vi "ConnectTestDisconnect.vi"() -> ()   [LabVIEW 2019]
panel:
  in  "DropPlate":u32=3229614090
  in  "Operation":T1(ring)
  in  "Autofocus":bool
  out "error out":errorcluster
  out "Image 2":T2(plugin-control)
  out "BestZvalue":dbl
  out "GantryXYUsingCamXY":cluster{"XmmGH":dbl, "YmmGH":dbl}
  in  "CamPixels":T3
  out "LogFilesPath":path
  in  "JoyStick":bool
  in  "GetHeightGauge Status":bool
  out "HeightGaugeTouch":bool
  out "SDofHeight(mm)":dbl format="%0.3f"
  out "MeanHeight(mm)":dbl format="%0.3f"
  in  "DistSensor":bool
  out "Position_XYZ":string
  in  "GetGantryXYZ":bool
  in  "DropTool":i32
  in  "PickPlate":u32=3233808386
  in  "PickTool":u32=3229614090
  in  "Z":dbl=50.0
  in  "PickDrop":bool
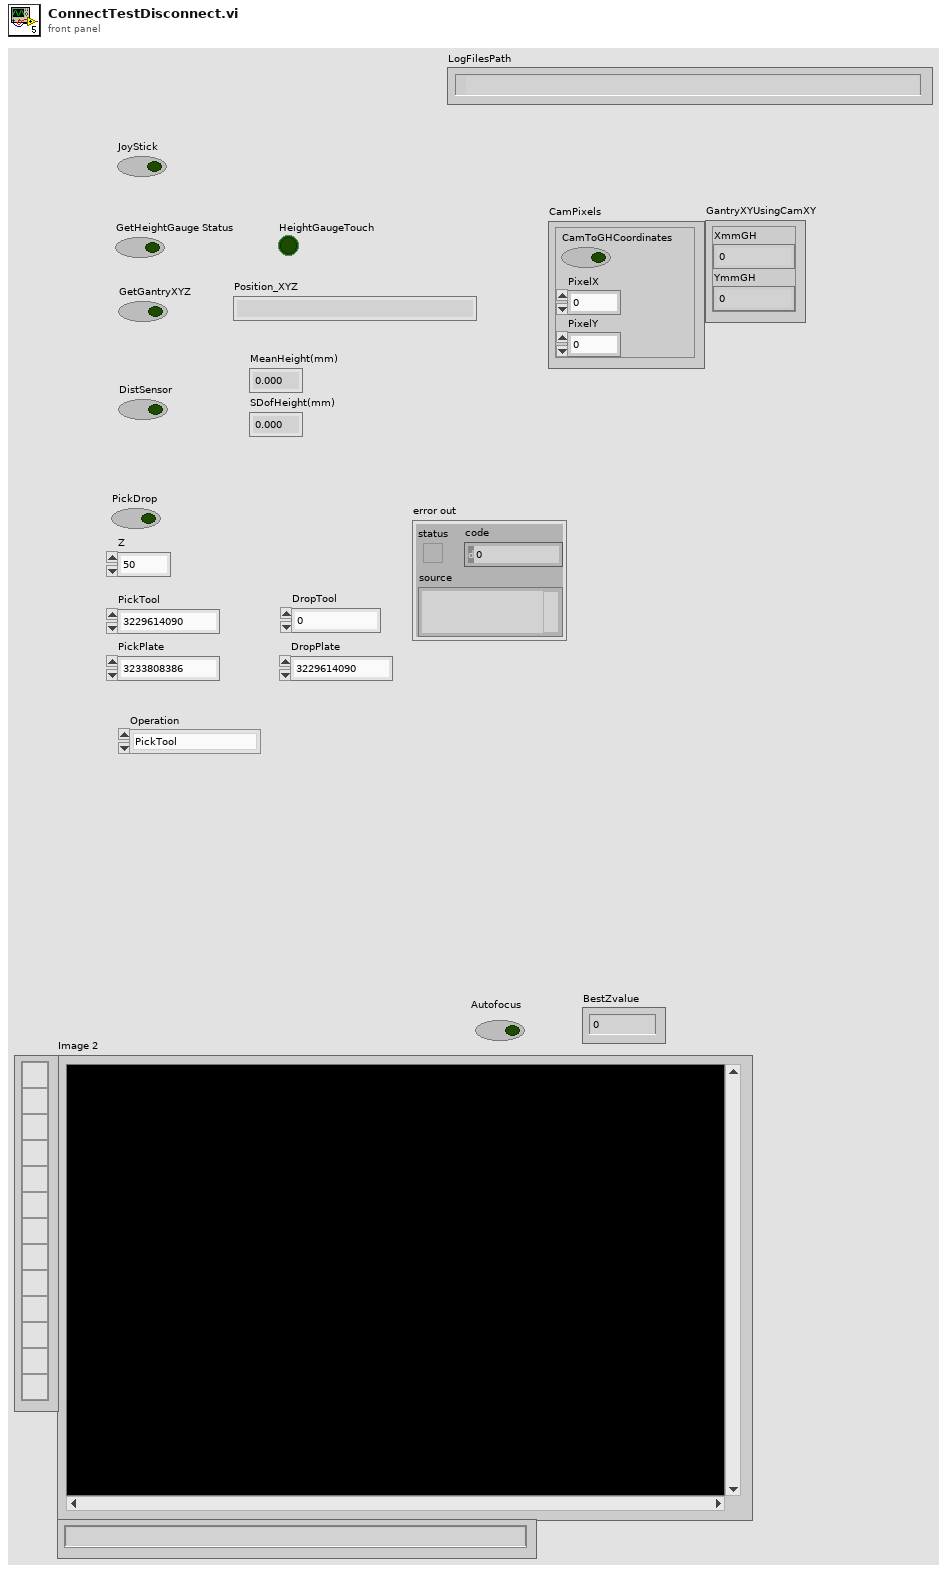
[diagram p1: front panel]
types:
  T1 = enum16{"PickTool", "PickPlate", "DropPlate", "DropTool"}
  T2 = typedef "IMAQ Image.ctl" = refnum<image>
  T3 = cluster{"CamToGHCoordinates":bool, "PixelX":dbl, "PixelY":dbl}
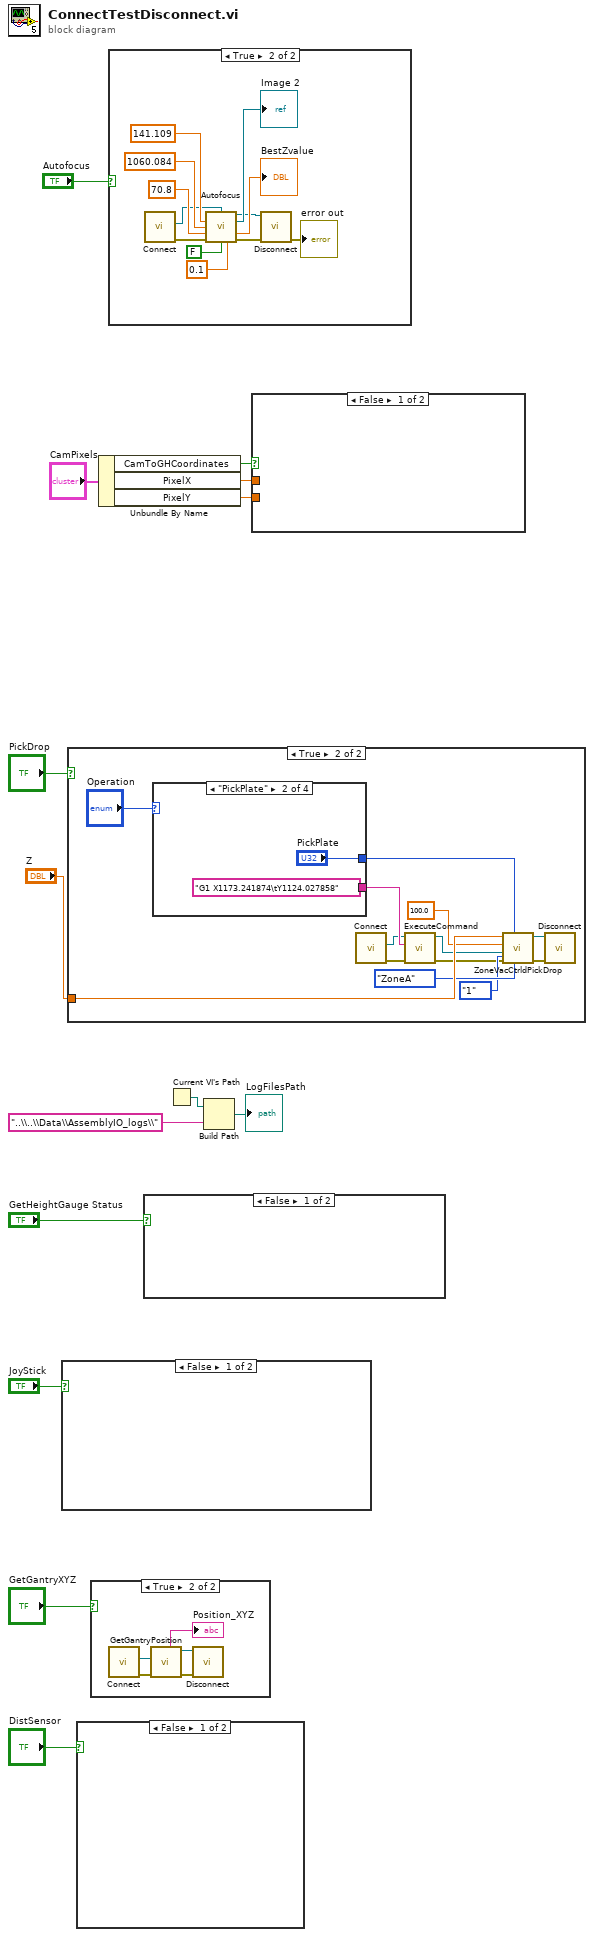
[diagram p0: block diagram]
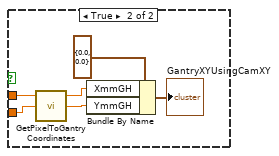
[diagram p3: hidden frame]
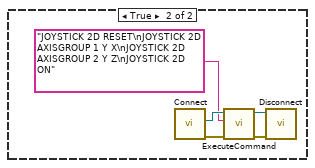
[diagram p4: hidden frame]
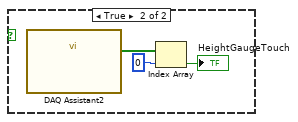
[diagram p5: hidden frame]
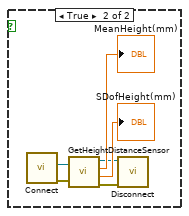
[diagram p6: hidden frame]
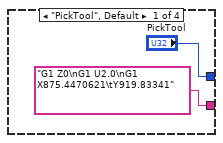
[diagram p9: hidden frame]
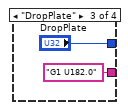
[diagram p10: hidden frame]
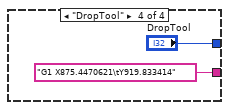
[diagram p11: hidden frame]
diagram:
  n1 = case shown="False" "JoyStick" {
    frame False {
    }
    frame True {
      n2 = call "Connect.vi"() -> ("error out"=w19:errorcluster, "controller"=w18:refnum<k24>)  [unwired: 10 in]
      n3 = call "ExecuteCommand.vi"("error in (no error)"=w19, "Command Code"="JOYSTICK 2D RESET\nJOYSTICK 2D AXISGROUP 1 Y X\nJOYSTICK 2D AXISGROUP 2 Y Z\nJOYSTICK 2D ON", "controller in"=w18) -> ("error out"=w16:errorcluster, "controller out"=w17:refnum<k24>)  [unwired: 6 in, 1 out]
      n4 = call "Disconnect.vi"("error in (no error)"=w16, "controller"=w17) -> ()  [unwired: 9 in, 1 out]
    }
  }
  n5 = case shown="True" "PickDrop" {
    tunnel: "Z" -> [_ w32]
    frame False {
    }
    frame True {
      n6 = case shown="\"PickPlate\"" "Operation" {
        tunnel: ["PickTool" "PickPlate" "DropPlate" "DropTool"] -> w25
        tunnel: ["G1 Z0\nG1 U2.0\nG1 X875.4470621\tY919.83341" "G1 X1173.241874\tY1124.027858" "G1 U182.0" "G1 X875.4470621\tY919.833414"] -> w23
        frame "PickTool", Default {
        }
        frame "PickPlate" {
        }
        frame "DropPlate" {
        }
        frame "DropTool" {
        }
      }
      n7 = call "Connect.vi"() -> ("error out"=w24:errorcluster, "controller"=w22:refnum<k24>)  [unwired: 10 in]
      n8 = call "ExecuteCommand.vi"("error in (no error)"=w24, "Command Code"=w23, "controller in"=w22) -> ("error out"=w21:errorcluster, "controller out"=w20:refnum<k24>)  [unwired: 6 in, 1 out]
      n9 = call "ZoneVacCtrldPickDrop.vi"("Position"=enum16{"1", "2"}."1", "Zone"=enum16{"ZoneA", "ZoneB", "ZoneC", "ZoneD"}."ZoneA", "VacuumState"=w25, "error in (no error)"=w21, "controller in"=w20, "Zspeed"=100.0, "Z"=w32) -> ("error out"=w27:errorcluster, "controller out"=w28:refnum<k24>)  [unwired: 3 in]
      n10 = call "Disconnect.vi"("error in (no error)"=w27, "controller"=w28) -> ()  [unwired: 9 in, 1 out]
    }
  }
  n11 = case shown="False" "DistSensor" {
    frame False {
    }
    frame True {
      n12 = call "Connect.vi"() -> ("error out"=w42:errorcluster, "controller"=w41:refnum<k24>)  [unwired: 10 in]
      n13 = call "GetHeightDistanceSensor.vi"("controller in"=w41, "error in (no error)"=w42) -> ("controller out"=w43:refnum<k24>, "MeanHeight(mm)"=→"MeanHeight(mm)":dbl, "SDofHeight(mm)"=→"SDofHeight(mm)":dbl, "error out"=w44:errorcluster)
      n14 = call "Disconnect.vi"("error in (no error)"=w44, "controller"=w43) -> ()  [unwired: 9 in, 1 out]
    }
  }
  n15 = case shown="True" "GetGantryXYZ" {
    frame False {
    }
    frame True {
      n16 = call "Connect.vi"() -> ("error out"=w49:errorcluster, "controller"=w50:refnum<k24>)  [unwired: 10 in]
      n17 = call "GetGantryPosition.vi"("error in (no error)"=w49, "Controller In"=w50) -> ("error out"=w48:errorcluster, "controller out"=w47:refnum<k24>, "Position_XYZ"=→"Position_XYZ":string)  [unwired: 3 in, 4 out]
      n18 = call "Disconnect.vi"("error in (no error)"=w48, "controller"=w47) -> ()  [unwired: 9 in, 1 out]
    }
  }
  n19 = Unbundle By Name("CamPixels") -> ("CamToGHCoordinates"=w4:bool, "PixelX"=w3:dbl, "PixelY"=w2:dbl)
  n20 = case shown="True" "Autofocus" {
    frame False {
    }
    frame True {
      n21 = call "Connect.vi"() -> ("error out"=w55:errorcluster, "controller"=w58:refnum<k24>)  [unwired: 10 in]
      n22 = call "Autofocus.vi"("controller in"=w58, "X"=141.109, "Y"=1060.084, "Z"=70.8, "error in (no error)"=w55, "AbortAutoFocus"=FALSE, "InitialStepSize"=0.1) -> ("controller out"=w57:refnum<k24>, "Image"=→"Image 2":T2, "BestZvalue"=→"BestZvalue":dbl, "error out"=w56:errorcluster)  [unwired: 4 in, 1 out]
      n23 = call "Disconnect.vi"("error in (no error)"=w56, "controller"=w57) -> ("error out"=→"error out":errorcluster)  [unwired: 9 in]
    }
  }
  n24 = case shown="False" "GetHeightGauge Status" {
    frame False {
    }
    frame True {
      n25 = call "DAQ Assistant2"() -> ("data"=w65:bool[])  [unwired: 17 in, 2 out]
      n26 = Index Array(array=w65, index=0) -> (element=→"HeightGaugeTouch":bool)
    }
  }
  n27 = Current VI's Path() -> (path=w7:path)
  n28 = Build Path(base path=w7, name or relative path="..\\..\\Data\\AssemblyIO_logs\\") -> (appended path=→"LogFilesPath":path)
  n29 = case shown="False" w4 {
    tunnel: w3 -> [_ w72]
    tunnel: w2 -> [_ w71]
    frame False {
    }
    frame True {
      n30 = call "GetPixelToGantryCoordinates.vi"("PixelY"=w71, "PixelX"=w72) -> ("YmmGH"=w69:dbl, "XmmGH"=w70:dbl)  [unwired: 1 in, 1 out]
      n31 = Bundle By Name(cluster=cluster{"XmmGH":dbl, "YmmGH":dbl} {"XmmGH"=0.0, "YmmGH"=0.0} ("Cluster 3"), "XmmGH"=w70, "YmmGH"=w69) -> (→"GantryXYUsingCamXY":cluster{"XmmGH":dbl, "YmmGH":dbl})
    }
  }
